vi "VerifyArrayVariant.vi"(8 "Generated Array":variant[](array[variant]), 9 "Array In":variant[](array[variant]), 10 "String To Append":string, 11 "Base":dbl format="%.2f") -> (3 "All Values Are Equal?":bool)   [LabVIEW 2012]
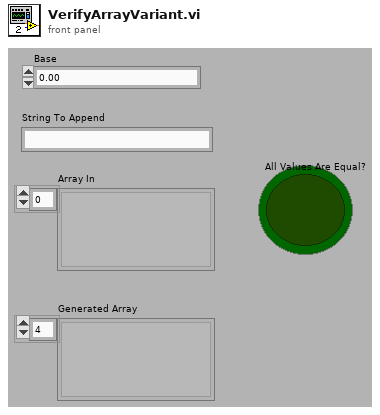
[diagram p1: front panel]
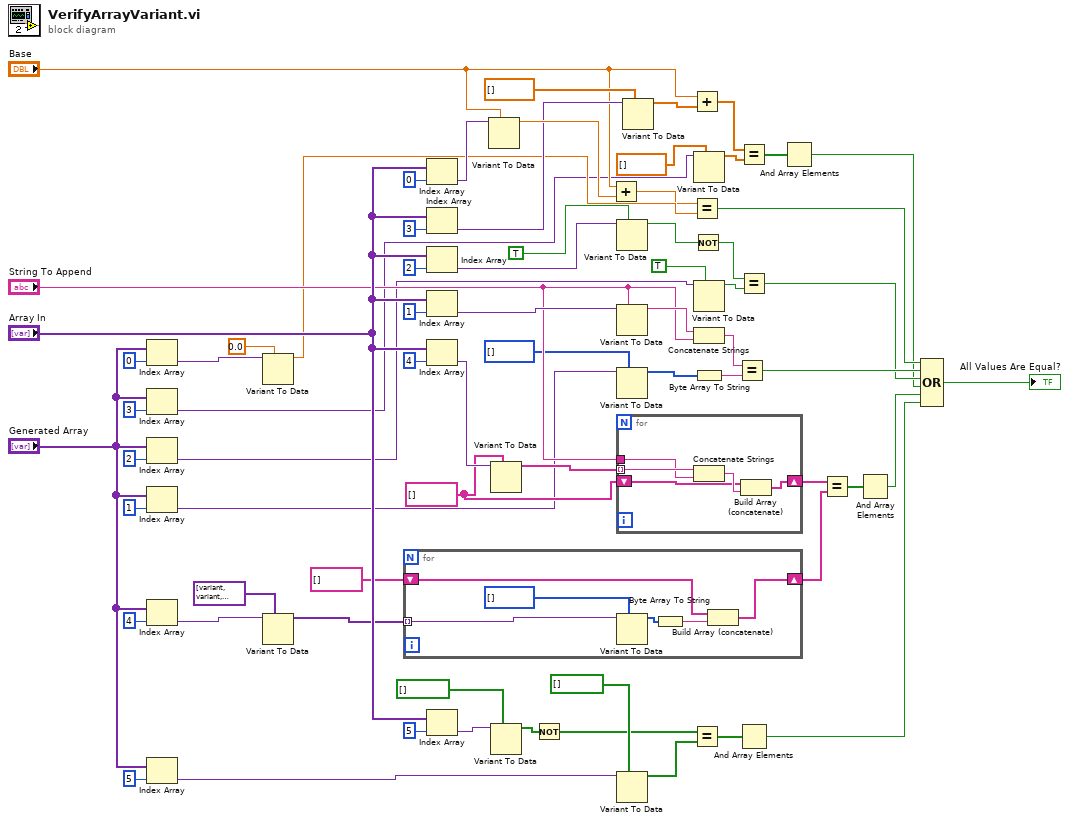
[diagram p0: block diagram]
diagram:
  w49 = string[] []
  n1 = Index Array(array="Generated Array", index=0) -> (element=w39:variant)
  n2 = Index Array(array="Generated Array", index=3) -> (element=w28:variant)
  n3 = Index Array(array="Generated Array", index=2) -> (element=w32:variant)
  n4 = Index Array(array="Generated Array", index=1) -> (element=w34:variant)
  n5 = Index Array(array="Generated Array", index=4) -> (element=w24:variant)
  n6 = Index Array(array="Generated Array", index=5) -> (element=w20:variant)
  n7 = Variant To Data(type=0.0 ("Base"), Variant=w39) -> (data=w37:dbl)  [unwired: 1 in, 1 out]
  n8 = Variant To Data(type=variant[] [variant, variant, variant, variant, variant, variant] ("Generated Array"), Variant=w24) -> (data=w2:variant[])  [unwired: 1 in, 1 out]
  n9 = for {
    tunnel: w2 -> [w75] mode=indexing
    shift-right: [w72] -> w1
    shift-left: string[] [] -> [w73]
    n10 = Variant To Data(type=u8[] [] ("x+y"), Variant=w75) -> (data=w71:u8[])  [unwired: 1 in, 1 out]
    n11 = Byte Array To String(unsigned byte array=w71) -> (string=w70:string)
    n12 = Build Array (concatenate)(w73, w70) -> (w72:string[])
  }
  n13 = Index Array(array="Array In", index=0) -> (element=w68:variant)
  n14 = Index Array(array="Array In", index=3) -> (element=w58:variant)
  n15 = Index Array(array="Array In", index=2) -> (element=w62:variant)
  n16 = Index Array(array="Array In", index=1) -> (element=w65:variant)
  n17 = Index Array(array="Array In", index=4) -> (element=w51:variant)
  n18 = Index Array(array="Array In", index=5) -> (element=w47:variant)
  n19 = Variant To Data(type="Base", Variant=w68) -> (data=w67:dbl)  [unwired: 1 in, 1 out]
  n20 = Variant To Data(type=w49, Variant=w51) -> (data=w50:string[])  [unwired: 1 in, 1 out]
  n21 = Variant To Data(type=bool[] [], Variant=w47) -> (data=w45:bool[])  [unwired: 1 in, 1 out]
  n22 = Not(x=w45) -> (.not. x?=w17:bool[])
  n23 = Add(x="Base", y=w67) -> (x+y=w36:dbl)
  n24 = Variant To Data(type=TRUE, Variant=w62) -> (data=w60:bool)  [unwired: 1 in, 1 out]
  n25 = Variant To Data(type="String To Append", Variant=w65) -> (data=w64:string)  [unwired: 1 in, 1 out]
  n26 = Variant To Data(type=u8[] [] ("x+y"), Variant=w34) -> (data=w33:u8[])  [unwired: 1 in, 1 out]
  n27 = for {
    tunnel: w50 -> [w80] mode=indexing
    shift-right: [w76] -> w23
    shift-left: w49 -> [w77]
    tunnel: "String To Append" -> [w79]
    n28 = Concatenate Strings(w80, w79) -> (w78:string)
    n29 = Build Array (concatenate)(w77, w78) -> (w76:string[])
  }
  n30 = Variant To Data(type=bool[] [], Variant=w20) -> (data=w18:bool[])  [unwired: 1 in, 1 out]
  n31 = Variant To Data(type=dbl[] [], Variant=w58) -> (data=w56:dbl[])  [unwired: 1 in, 1 out]
  n32 = Add(x="Base", y=w56) -> (x+y=w25:dbl[])
  n33 = Equal?(x=w36, y=w37) -> (x = y?=w13:bool)
  n34 = Equal?(x=w17, y=w18) -> (x = y?=w14:bool[])
  n35 = Not(x=w60) -> (.not. x?=w30:bool)
  n36 = Variant To Data(type=dbl[] [] ("x+y"), Variant=w28) -> (data=w26:dbl[])  [unwired: 1 in, 1 out]
  n37 = Variant To Data(type=TRUE, Variant=w32) -> (data=w29:bool)  [unwired: 1 in, 1 out]
  n38 = Concatenate Strings(w64, "String To Append") -> (w35:string)
  n39 = Byte Array To String(unsigned byte array=w33) -> (string=w5:string)
  n40 = Equal?(x=w35, y=w5) -> (x = y?=w12:bool)
  n41 = Equal?(x=w25, y=w26) -> (x = y?=w16:bool[])
  n42 = Equal?(x=w30, y=w29) -> (x = y?=w11:bool)
  n43 = And Array Elements(Boolean array=w14) -> (logical AND=w8:bool)
  n44 = And Array Elements(Boolean array=w16) -> (logical AND=w10:bool)
  n45 = Equal?(x=w23, y=w1) -> (x = y?=w15:bool[])
  n46 = And Array Elements(Boolean array=w15) -> (logical AND=w9:bool)
  n47 = Compound Arithmetic op=OR(w13, w12, w11, w10, w9, w8) -> (→"All Values Are Equal?":bool)
